vi "PXF4_get_PV_param.vi"(8 "error in":errorcluster, 11 "Modbus Master in":refnum<class "Modbus Master.lvclass">) -> (0 "error out":errorcluster, 3 "Modbus Master out":refnum<class "Modbus Master.lvclass">)   [LabVIEW 2019]
uses:
  <vilib>/NI/Modbus Library/API/Master/Modbus Master.lvclass
panel:
  out "decimal point position":u16
  out "PV input upper limit":u16
  out "PV input lower limit":u16
  out "unit":u16
  out "PV input type":u16
  out "register values":u16[](array[numeric])
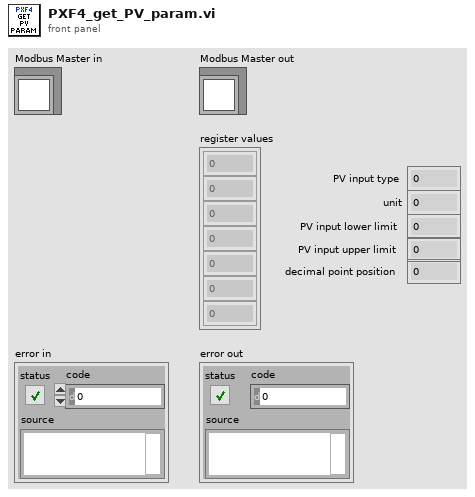
[diagram p1: front panel]
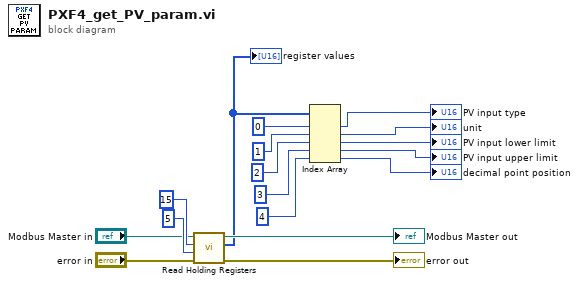
[diagram p0: block diagram]
diagram:
  n1 = call-dynamic "Read Holding Registers.vi"("error in"="error in", "number of inputs"=u16 5, "starting address"=u16 15, "Modbus master in"="Modbus Master in") -> ("error out"=→"error out":errorcluster, "register values"=w11:u16[], "Modbus master out"=→"Modbus Master out":refnum<class "Modbus Master.lvclass">)  [unwired: 5 in]
  "register values" <- w11
  n2 = Index Array(array=w11, index #1=0 ("index"), index #2=1 ("index"), index #3=2 ("index"), index #4=3 ("index"), index #5=4 ("index")) -> (element #1=→"PV input type":u16, element #2=→"unit":u16, element #3=→"PV input lower limit":u16, element #4=→"PV input upper limit":u16, element #5=→"decimal point position":u16)
